vi "end timer Write.vi"(4 "error in (no error)":errorcluster, 5 "Value":bool, 6 "Container State":T4, 7 "Display State In":T1) -> (0 "error out":errorcluster, 3 "Display State Out":T1)   [LabVIEW 2019, in "Heating.lvlib" / "YQ2.xctl"]
uses:
  YQ2.xctl
  <vilib>/_xctls/Container State.ctl
  State.ctl
  Y_state.ctl
  Y_controlState.ctl
  <vilib>/_xctls/XControlSupport.lvlib
  Heating.lvlib
panel:
  # "Replace the Value Control below with a Control of desired type.\nDo not remove this Control or the others from the connector pane.\nDo not change the connector pane pattern.\nThe Value control should always be the third terminal from top on the input side in the connector pane."
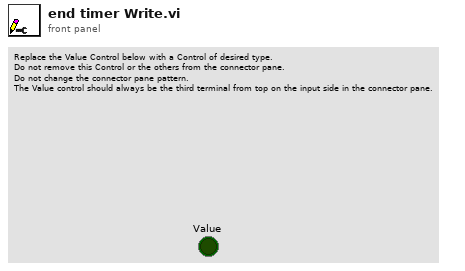
[diagram p1: front panel]
types:
  T1 = typedef "Heating.lvlib/YQ2.xctl/State.ctl" = cluster{"Y_State":cluster{"connect":bool, "Y_State":T2, "Y":dbl}, "Write":bool, "button state":T3, "reset_timer":bool, "load_timer":bool, "end_timer":bool}
  T2 = typedef "Heating.lvlib/Y_state.ctl" = enum8{"initialize", "alarm", "min", "stop", "hand", "auto", "max"}
  T3 = typedef "Heating.lvlib/YQ2.xctl/Y_controlState.ctl" = enum16{"init", "not connect", "alarm", "min", "stop", "hand", "value change", "auto", "max"}
  T4 = typedef "XControlSupport.lvlib/Container State.ctl" = cluster{"Indicator?":bool, "Run Mode?":bool, " Refnum":refnum<vi>}
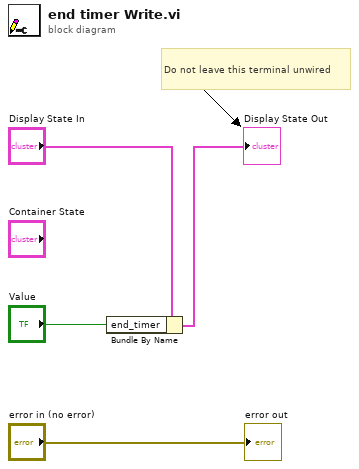
[diagram p0: block diagram]
diagram:
  # "Do not leave this terminal unwired"
  n1 = Bundle By Name(cluster="Display State In", "end_timer"="Value") -> (→"Display State Out":T1)
  "error out" <- "error in (no error)"
